vi "Trial3.vi"() -> ()   [LabVIEW 2013]
doc: "This example shows how to acquire measurements and save those measurements to a file."
panel:
  in  "Output File":path=path "c:/polaris.txt"
  out "Current Transformations":T1(array[cluster])
  in  "Track Stray Markers? (F:No)":bool
  in  "VISA resource name":refnum<visa-resource-name>="COM1"
  in  "Reset? (T:Yes)":bool=TRUE
  in  "Track Outside Measurement Volume? (F:No)":bool
  in  "Location of ROM File for Tool":path=path "C:/Program Files/Northern Digital Inc/8700248.rom"
  in  "Serial Configuration":T2={"Baud Rate (9600)"=9600, "Flow Control (0:None)"=0, "Parity"=0, "Data Bits"=8, "Stop Bits"=10} {"Stop Bits" items=["1.0"=10, "2.0"=20]; "Parity" items=["None", "Odd", "Even"]; "Flow Control (0:None)" items=["None", "XON/XOFF"]; "Baud Rate (9600)" items=["9600"=9600, "14.4k"=14400, "19.2k"=19200, "38.4k"=38400, "57.6k "=57600, "115.2k"=115200]}
  in  "STOP":bool
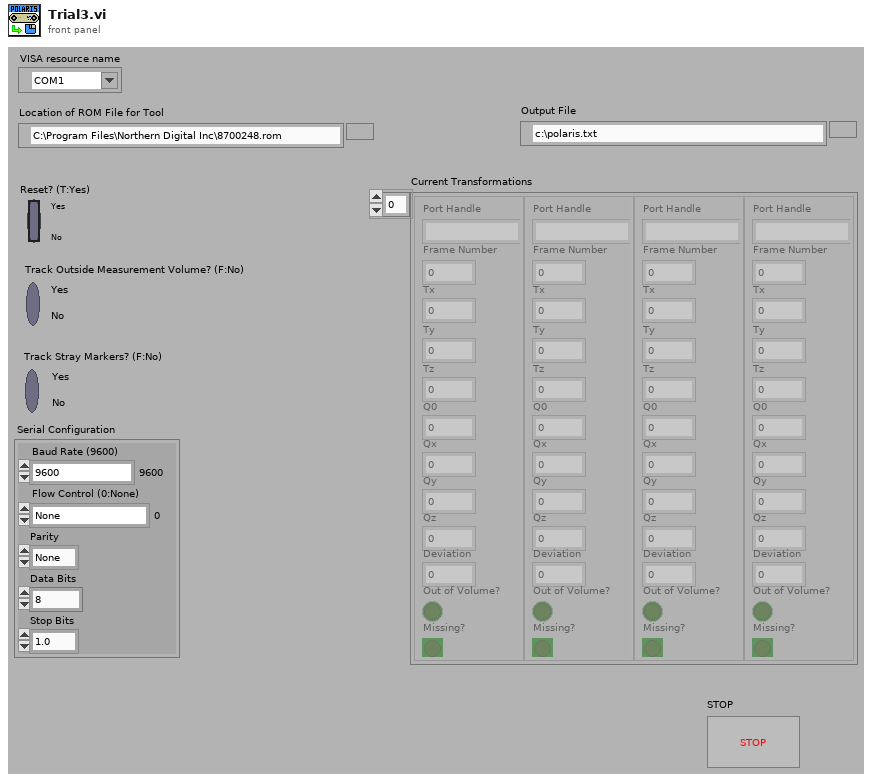
[diagram p1: front panel]
types:
  T1 = cluster{"Port Handle":string, "Frame Number":u32, "Tx":dbl, "Ty":dbl, "Tz":dbl, "Q0":dbl, "Qx":dbl, "Qy":dbl, "Qz":dbl, "Deviation":dbl, "Missing?":bool, "Out of Volume?":bool}[]
  T2 = cluster{"Baud Rate (9600)":u32, "Flow Control (0:None)":u16, "Parity":u16, "Data Bits":u16, "Stop Bits":u16}
  T3 = enum16{"open", "open or create", "create or replace", "create", "open (read only)"}
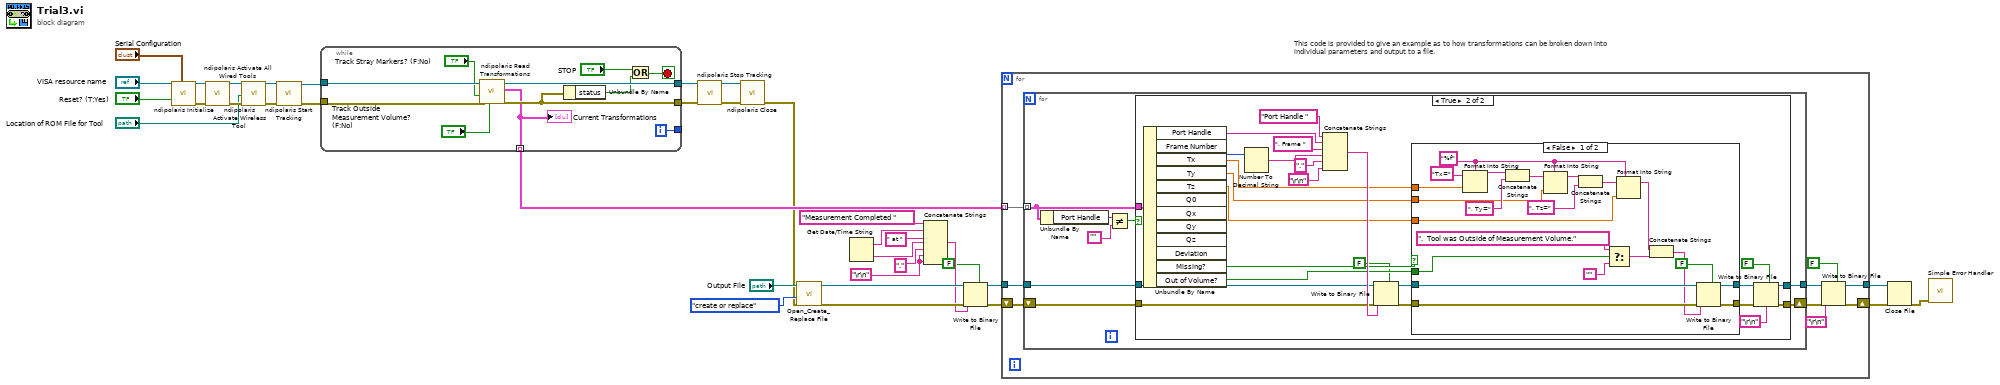
[diagram p0: block diagram]
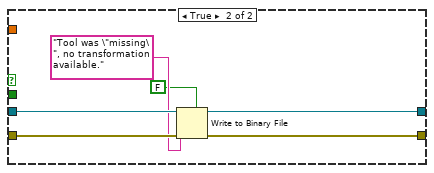
[diagram p3: hidden frame]
diagram:
  w4 = "\r\n"
  # "This code is provided to give an example as to how transformations can be broken down into\nindividual parameters and output to a file."
  n1 = call <instrlib>:"ndipolaris Initialize.vi"("Serial Configuration"="Serial Configuration", "Reset? (T: Yes)"="Reset? (T:Yes)", "VISA resource name"="VISA resource name") -> ("error out"=w27:errorcluster, "VISA resource name out"=w28:refnum<visa-resource-name>)  [unwired: 7 in]
  n2 = call <instrlib>:"ndipolaris Activate All Wired Tools.vi"("error in (no error)"=w27, "VISA resource name"=w28) -> ("error out"=w34:errorcluster, "VISA resource out"=w35:refnum<visa-resource-name>)  [unwired: 7 in, 1 out]
  n3 = call <instrlib>:"ndipolaris Activate Wireless Tool.vi"("error in (no error)"=w34, "Location of ROM File for Tool"="Location of ROM File for Tool", "VISA resource name"=w35) -> ("error out"=w31:errorcluster, "VISA resource out"=w32:refnum<visa-resource-name>)  [unwired: 6 in, 1 out]
  n4 = call <instrlib>:"ndipolaris Start Tracking.vi"("error in (no error)"=w31, "VISA resource name"=w32) -> ("error out"=w29:errorcluster, "VISA resource out"=w30:refnum<visa-resource-name>)  [unwired: 8 in]
  n5 = while {
    tunnel: w30 -> [w46]
    tunnel: w29 -> [w45]
    tunnel: [w39] -> _
    tunnel: [w42] -> w25
    tunnel: [w41] -> w24
    tunnel: [w36] -> w19 mode=indexing
    i -> [w39]
    stop <- w44 stop-if-true
    n6 = call <instrlib>:"ndipolaris Read Transformations.vi"("Track Outside Measurement Volume? (F:No)"="Track Outside Measurement Volume? (F:No)", "error in (no error)"=w45, "Track Stray Markers? (F:No)"="Track Stray Markers? (F:No)", "VISA resource name"=w46) -> ("error out"=w41:errorcluster, "Transformations"=w36:T1, "VISA resource out"=w42:refnum<visa-resource-name>)  [unwired: 4 in, 1 out]
    "Current Transformations" <- w36
    n7 = Unbundle By Name(w41) -> ("status"=w40:bool)
    n8 = Or(x="STOP", y=w40) -> (x .or. y?=w44:bool)
  }
  n9 = call <instrlib>:"ndipolaris Stop Tracking.vi"("error in (no error)"=w24, "VISA resource name"=w25) -> ("error out"=w21:errorcluster, "VISA resource out"=w22:refnum<visa-resource-name>)  [unwired: 8 in]
  n10 = call <instrlib>:"ndipolaris Close.vi"("error in (no error)"=w21, "VISA resource name"=w22) -> ("error out"=w3:errorcluster)  [unwired: 9 in]
  n11 = call <vilib>:"Open_Create_Replace File.vi"("error in (no error)"=w3, "function (open:0)"=T3."create or replace", "file path"="Output File") -> ("error out"=w15:errorcluster, "refnum"=w16:refnum<file>)  [unwired: 5 in, 2 out]
  n12 = Get Date/Time String() -> (date string=w13:string, time string=w11:string)  [unwired: 3 in]
  n13 = Concatenate Strings("Measurement Completed ", w13, " at ", w11, "." ("string"), w4, w4) -> (w10:string)
  n14 = Write to Binary File(file (use dialog)=w16, data=w10, error in=w15, 5:FALSE ("prepend array or string size? (T)")) -> (refnum out=w9:refnum<file>, error out=w8:errorcluster)  [unwired: 2 in, 1 out]
  n15 = for {
    tunnel: w19 -> [w55] mode=indexing
    tunnel: w9 -> [w54]
    shift-right: [w49] -> w6
    shift-left: w8 -> [w53]
    tunnel: [w50] -> w7
    n16 = for {
      tunnel: w55 -> [w59] mode=indexing
      tunnel: w54 -> [w63]
      tunnel: [w61] -> w51
      shift-right: [w60] -> w52
      shift-left: w53 -> [w62]
      n17 = Unbundle By Name(w59) -> ("Port Handle"=w58:string)
      n18 = Not Equal?(x=w58, y="") -> (x != y?=w57:bool)
      n19 = case shown="True" w57 {
        tunnel: w59 -> [_ w90]
        tunnel: w63 -> [w65 w82]
        tunnel: w62 -> [w64 w81]
        tunnel: [w65 w71] -> w61
        tunnel: [w64 w70] -> w60
        frame False {
        }
        frame True {
          n20 = Unbundle By Name(w90) -> ("Port Handle"=w84:string, "Frame Number"=w89:u32, "Tx"=w76:dbl, "Ty"=w75:dbl, "Tz"=w74:dbl, "Missing?"=w77:bool, "Out of Volume?"=w68:bool)  [unwired: 5 out]
          n21 = Number To Decimal String(number=w89) -> (decimal integer string=w87:string)  [unwired: 1 in]
          n22 = Concatenate Strings("Port Handle " ("string"), w84, ", Frame ", w87, "." ("string"), "\r\n") -> (w83:string)
          n23 = Write to Binary File(file (use dialog)=w82, data=w83, error in=w81, 5:FALSE ("prepend array or string size? (T)")) -> (refnum out=w79:refnum<file>, error out=w78:errorcluster)  [unwired: 2 in, 1 out]
          n24 = case shown="False" w77 {
            tunnel: w79 -> [w99 w118]
            tunnel: w78 -> [w98 w117]
            tunnel: [w101 w115] -> w72
            tunnel: [w100 w114] -> w73
            tunnel: w76 -> [w111 _]
            tunnel: w75 -> [w107 _]
            tunnel: w74 -> [w102 _]
            tunnel: w68 -> [w95 _]
            frame False {
              w104 = "%f" ("format string")
              n25 = Format Into String(format string=w104, initial string="Tx=", w111) -> (resulting string=w110:string)  [unwired: 1 in, 1 out]
              n26 = Concatenate Strings(w110, ", Ty=") -> (w108:string)
              n27 = Format Into String(format string=w104, initial string=w108, w107) -> (resulting string=w106:string)  [unwired: 1 in, 1 out]
              n28 = Concatenate Strings(w106, ", Tz=") -> (w105:string)
              n29 = Select(t=".  Tool was Outside of Measurement Volume.", s=w95, f="") -> (s? t:f=w92:string)
              n30 = Format Into String(format string=w104, initial string=w105, w102) -> (resulting string=w97:string)  [unwired: 1 in, 1 out]
              n31 = Concatenate Strings(w97, w92) -> (w96:string)
              n32 = Write to Binary File(file (use dialog)=w99, data=w96, error in=w98, 5:FALSE ("prepend array or string size? (T)")) -> (refnum out=w101:refnum<file>, error out=w100:errorcluster)  [unwired: 2 in, 1 out]
            }
            frame True {
              n33 = Write to Binary File(file (use dialog)=w118, data="Tool was \"missing\", no transformation available.", error in=w117, 5:FALSE ("prepend array or string size? (T)")) -> (refnum out=w115:refnum<file>, error out=w114:errorcluster)  [unwired: 2 in, 1 out]
            }
          }
          n34 = Write to Binary File(file (use dialog)=w72, data="\r\n", error in=w73, 5:FALSE ("prepend array or string size? (T)")) -> (refnum out=w71:refnum<file>, error out=w70:errorcluster)  [unwired: 2 in, 1 out]
        }
      }
    }
    n35 = Write to Binary File(file (use dialog)=w51, data="\r\n", error in=w52, 5:FALSE ("prepend array or string size? (T)")) -> (refnum out=w50:refnum<file>, error out=w49:errorcluster)  [unwired: 2 in, 1 out]
  }
  n36 = Close File(refnum=w7, error in=w6) -> (error out=w2:errorcluster)  [unwired: 1 out]
  n37 = call <vilib>:"Simple Error Handler.vi"("error in (no error)"=w2) -> ()  [unwired: 4 in, 5 out]
